vi "Test Report By Month_ABB.vi"() -> ()   [LabVIEW 2017]
uses:
  <vilib>/Utility/miscctls.llb/LVDateTimeRec.ctl
  ABB global.vi
panel:
  in  "Print":bool
  in  "Quit":bool
  in  "Go":bool
  in  "To":timestamp format="%<%m/%Y>T"
  in  "From":timestamp format="%<%m/%Y>T"
  out "XY Graph":cluster{u64[], i32[]}(graph)
  in  "Motors Tested":i32(listbox)
  # "Motors Tested"
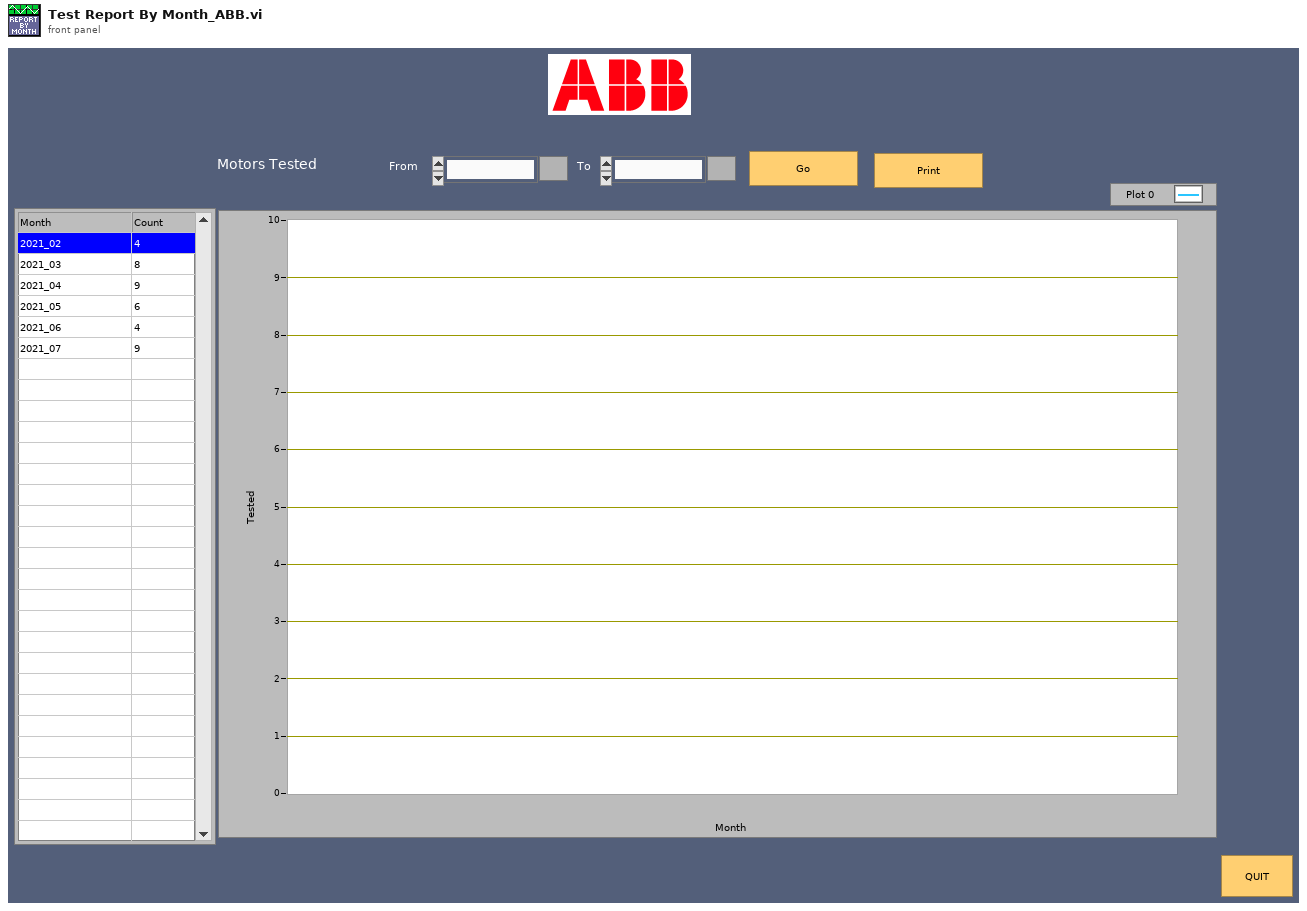
[diagram p1: front panel]
types:
  T1 = typedef "LVDateTimeRec.ctl" = cluster{"fractional second":dbl, "second":i32, "minute":i32, "hour":i32, "day of month":i32, "month":i32, "year":i32, "day of week":i32, "day of year":i32, "DST":i32}
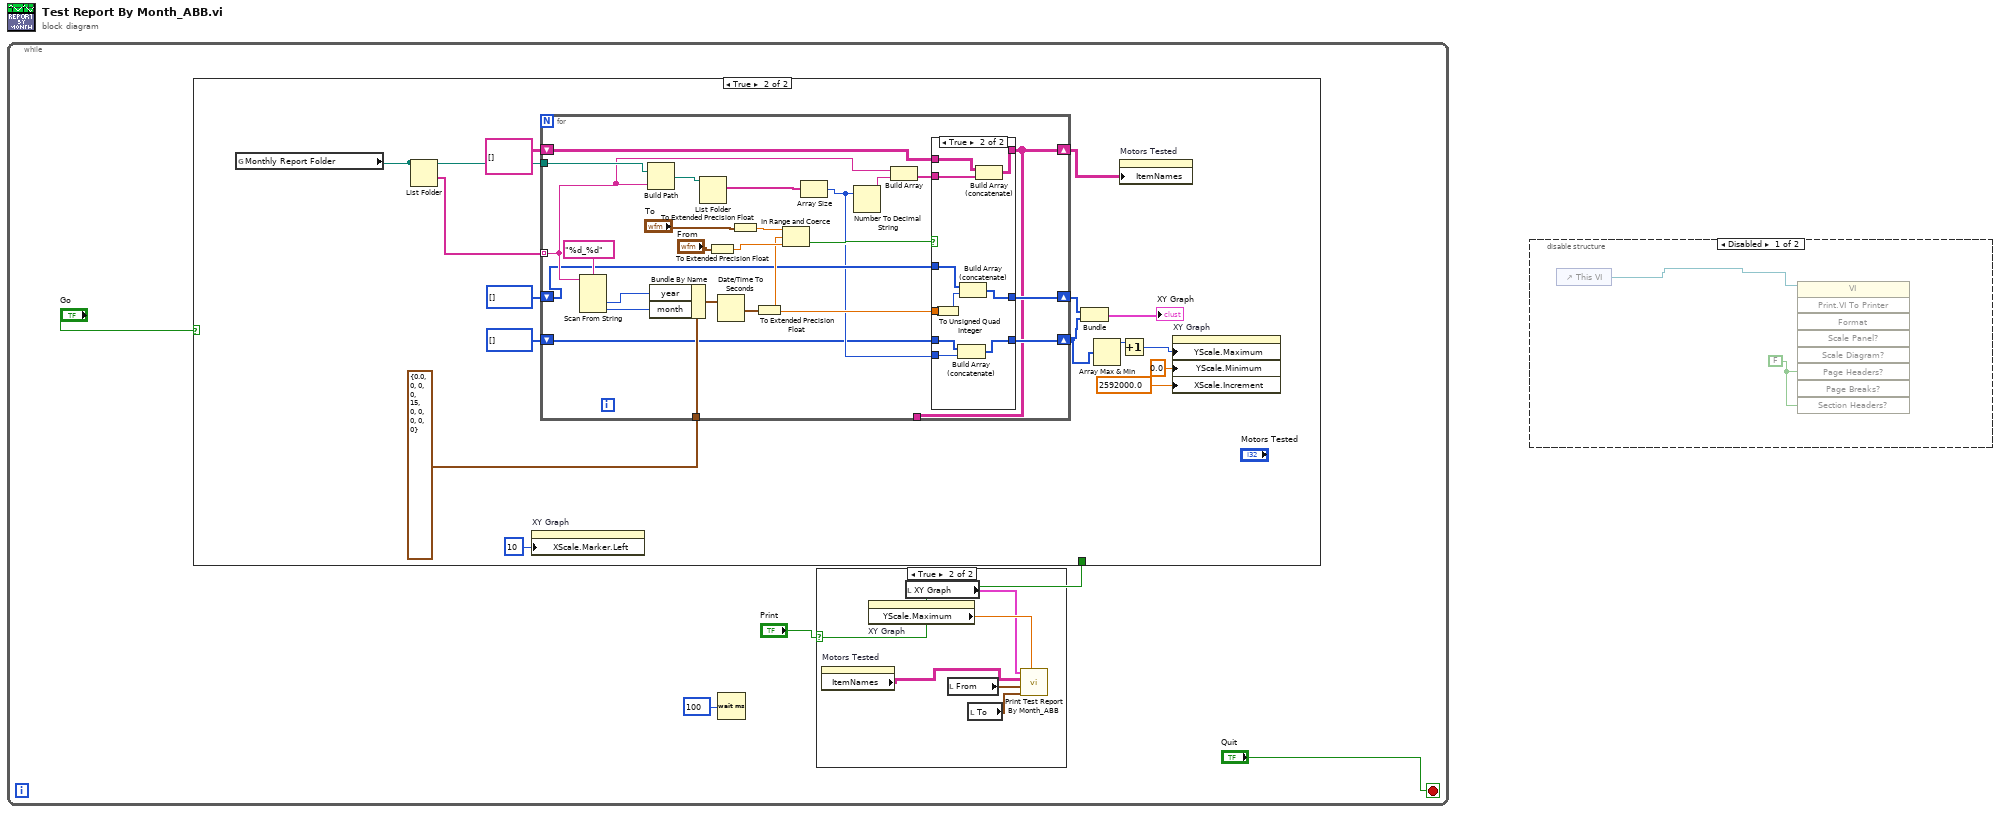
[diagram p0: block diagram]
diagram:
  n1 = while {
    stop <- "Quit" stop-if-true
    n2 = case shown="True" "Go" {
      tunnel: "Print" -> [_ _]
      frame False {
      }
      frame True {
        n3 = global read "ABB global.vi" "Monthly Report Folder"() -> (w23:path)
        n4 = List Folder(path=w23) -> (folder names=w24:string[])  [unwired: 3 in, 3 out]
        n5 = property on="XY Graph" class="XYGraph (strict)"("XScale.Marker.Left"=10 ("X Scale.Marker.Position:Left")) -> ()  [unwired: 2 in, 2 out]
        n6 = for {
          tunnel: w24 -> [w45] mode=indexing
          tunnel: w23 -> [w49]
          tunnel: T1 {"fractional second"=0.0, "second"=0, "minute"=0, "hour"=0, "day of month"=15, "month"=0, "year"=0, "day of week"=0, "day of year"=0, "DST"=0} ("date time rec") -> [w41]
          shift-right: [w31] -> w20
          shift-left: u64[] [] -> [w30]
          shift-right: [w28] -> w19
          shift-left: i32[] [] -> [w27]
          shift-right: [w25] -> w12
          shift-left: string[][] [] -> [w33]
          tunnel: [w25] -> _
          n7 = Scan From String(format string="%d_%d", input string=w45) -> (output 1=w43:i32, output 2=w26:i32)  [unwired: 4 in, 3 out]
          n8 = Build Path(base path=w49, name or relative path=w45) -> (appended path=w48:path)
          n9 = Bundle By Name(cluster=w41, "year"=w43, "month"=w26) -> (w40:T1)
          n10 = List Folder(path=w48) -> (filenames=w47:string[])  [unwired: 3 in, 3 out]
          n11 = To Extended Precision Float(1:"From") -> (0:w38:ext)
          n12 = Date/Time To Seconds(2:w40) -> (0:w42:timestamp)  [unwired: 1 in]
          n13 = To Extended Precision Float(1:"To") -> (0:w36:ext)
          n14 = To Extended Precision Float(1:w42) -> (0:w32:ext)
          n15 = In Range and Coerce(upper limit=w36, x=w32, lower limit=w38) -> (In Range?=w35:bool)  [unwired: 1 out]
          n16 = Array Size(array=w47) -> (size(s)=w29:i32)
          n17 = Number To Decimal String(number=w29) -> (decimal integer string=w46:string)  [unwired: 1 in]
          n18 = Build Array(w45, w46) -> (w34:string[])
          n19 = case shown="True" w35 {
            tunnel: w34 -> [_ w62]
            tunnel: [w52 w61] -> w25
            tunnel: w33 -> [w52 w60]
            tunnel: w32 -> [_ w58]
            tunnel: [w51 w57] -> w31
            tunnel: w30 -> [w51 w56]
            tunnel: w29 -> [_ w55]
            tunnel: [w50 w54] -> w28
            tunnel: w27 -> [w50 w53]
            frame False {
            }
            frame True {
              n20 = To Unsigned Quad Integer(1:w58) -> (0:w59:u64)
              n21 = Build Array (concatenate)(w53, w55) -> (w54:i32[])
              n22 = Build Array (concatenate)(w56, w59) -> (w57:u64[])
              n23 = Build Array (concatenate)(w60, w62) -> (w61:string[][])
            }
          }
        }
        n24 = Bundle(w20, w19) -> (→"XY Graph":cluster{u64[], i32[]})  [unwired: 1 in]
        n25 = Array Max & Min(array=w19) -> (max value=w17:i32)  [unwired: 3 out]
        n26 = property on="Motors Tested" class="MCListbox (strict)"("ItemNames"=w12) -> ()  [unwired: 2 in, 2 out]
        n27 = Increment(x=w17) -> (x+1=w10:i32)
        n28 = property on="XY Graph" class="XYGraph (strict)"("YScale.Maximum"=w10, "YScale.Minimum"=0.0 ("Y Scale.Range:Minimum"), "XScale.Increment"=2592000.0 ("X Scale.Range:Increment")) -> ()  [unwired: 2 in, 2 out]
      }
    }
    n29 = Wait (ms)(milliseconds to wait=u32 100) -> ()  [unwired: 1 out]
    n30 = case shown="True" "Print" {
      frame False {
      }
      frame True {
        n31 = property on="Motors Tested" class="MCListbox (strict)"() -> ("ItemNames"=w7:string[][])  [unwired: 2 in, 2 out]
        n32 = property on="XY Graph" class="XYGraph (strict)"() -> ("YScale.Maximum"=w6:dbl)  [unwired: 2 in, 2 out]
        n33 = local read "XY Graph"() -> (w5:cluster{u64[], i32[]})
        n34 = local read "From"() -> (w8:timestamp)
        n35 = local read "To"() -> (w9:timestamp)
        n36 = call "Print Test Report By Month_ABB.vi"("Y Scale.Range:Maximum"=w6, "To"=w9, "From"=w8, "List"=w7, "XY Graph"=w5) -> ()  [unwired: 7 in]
      }
    }
  }
  n37 = disable-structure shown="Disabled" {
    frame Disabled {
      w64 = FALSE ("Page Headers?")
      n38 = control-ref of="This VI"() -> (w63:refnum<vi>)
      n39 = invoke class="VI" method="Print.VI To Printer"(reference=w63, "Page Headers?"=w64, "Section Headers?"=w64) -> ()  [unwired: 6 in, 9 out]
    }
    frame Enabled {
    }
  }
